vi "Send-priority-message.vi"(8 "error in (no error)":errorcluster, 11 "Client in":T1) -> (0 "error out":errorcluster, 3 "Client out":T1)   [LabVIEW 2013, in "Module-communication.lvlib" / "Client.lvclass"]
uses:
  Client.lvclass
  Object-reference.ctl
  Messages/Message.lvclass
  Client.lvclass/Client.ctl
panel:
  in  "Receivers":string[](array[string])
  in  "Message":refnum<class "Message.lvclass">
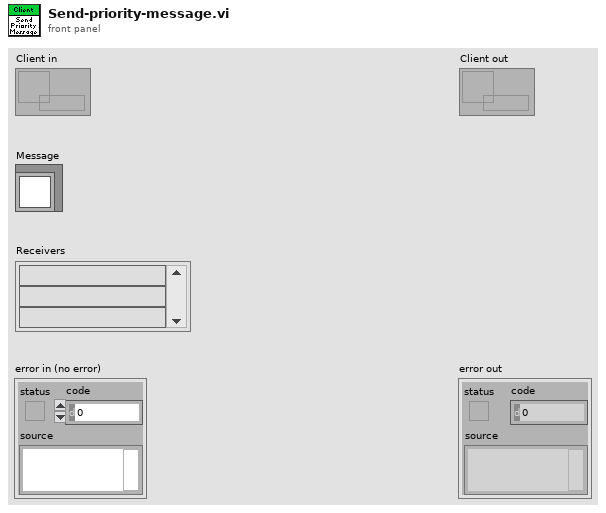
[diagram p1: front panel]
types:
  T1 = typedef "Module-communication.lvlib/Client.lvclass/Object-reference.ctl" = refnum<data-value>
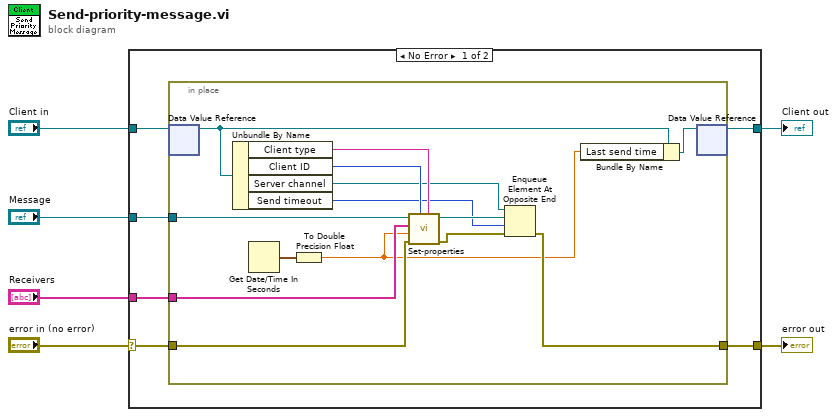
[diagram p0: block diagram]
diagram:
  n1 = case shown="No Error" "error in (no error)" {
    selector: "error in (no error)" -> [w8 w28]
    tunnel: [w7 w28] -> w5
    tunnel: [w9 w27] -> w3
    tunnel: "Client in" -> [w10 w27]
    tunnel: "Message" -> [w12 _]
    tunnel: "Receivers" -> [w11 _]
    frame No Error {
      n2 = in-place {
        in-place-border: w12 -> [w26]
        in-place-border: w11 -> [w25]
        in-place-border: w8 -> [w23]
        in-place-border: [w18] -> w7
        n3 = in-place-dvr #1(w10) -> (w15:refnum<class "Client.lvclass">)  [unwired: 1 out]
        n4 = Unbundle By Name(w15) -> ("Client type"=w21:string, "Client ID"=w22:i32, "Server channel"=w16:refnum<queue>, "Send timeout"=w17:i32)
        n5 = Get Date/Time In Seconds() -> (seconds since 1Jan1904=w24:timestamp)
        n6 = To Double Precision Float(number=w24) -> (double precision float=w13:dbl)
        n7 = call "Set-properties.vi"("Sender type"=w21, "Sender ID"=w22, "error in (no error)"=w23, "Send time"=w13, "Receivers"=w25, "Message in"=w26) -> ("error out"=w19:errorcluster, "Message out"=w20:refnum<class "Message.lvclass">)  [unwired: 4 in]
        n8 = Enqueue Element At Opposite End(queue=w16, element=w20, timeout in ms (-1)=w17, error in (no error)=w19) -> (error out=w18:errorcluster)  [unwired: 2 out]
        n9 = Bundle By Name(cluster=w15, "Last send time"=w13) -> (w14:refnum<class "Client.lvclass">)
        n10 = in-place-dvr #1(w14) -> (w9:T1)  [unwired: 1 out]
      }
    }
    frame Error {
    }
  }
  "error out" <- w5
  "Client out" <- w3
